vi "vector_cord2vect.vi"(11 "Coordinate":cluster{"X":dbl, "Y":dbl}) -> (3 "Vector":cluster{"R":dbl, "theta":dbl})   [LabVIEW 2011]
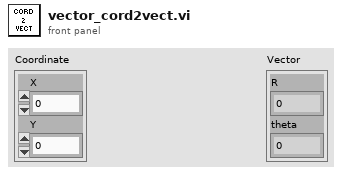
[diagram p1: front panel]
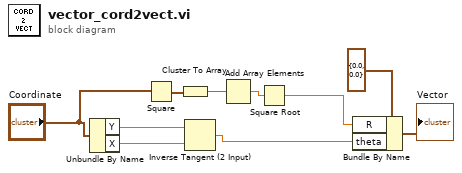
[diagram p0: block diagram]
diagram:
  n1 = Unbundle By Name("Coordinate") -> ("Y"=w3:dbl, "X"=w2:dbl)
  n2 = Square(x="Coordinate") -> (x^2=w9:cluster{"X":dbl, "Y":dbl})
  n3 = Cluster To Array(cluster=w9) -> (array=w8:dbl[])
  n4 = Inverse Tangent (2 Input)(1:w2, 2:w3) -> (0:w1:dbl)
  n5 = Add Array Elements(numeric array=w8) -> (sum=w7:dbl)
  n6 = Square Root(x=w7) -> (sqrt(x)=w4:dbl)
  n7 = Bundle By Name(cluster=cluster{"R":dbl, "theta":dbl} {"R"=0.0, "theta"=0.0} ("Vector"), "R"=w4, "theta"=w1) -> (→"Vector":cluster{"R":dbl, "theta":dbl})
